vi "Write Message.vi"(8 "error in (no error)":errorcluster, 10 "Message":string, 11 "Printf_Msg_General in":refnum<class "LV_Printf Msg.lvclass">) -> (0 "error out":errorcluster, 3 "Printf_Msg_General out":refnum<class "LV_Printf Msg.lvclass">)   [LabVIEW 2013, in "SET_Printf.lvlib" / "LV_Printf Msg.lvclass"]
uses:
  LV_Printf Msg.lvclass
  LV_Printf Msg.lvclass/LV_Printf Msg.ctl
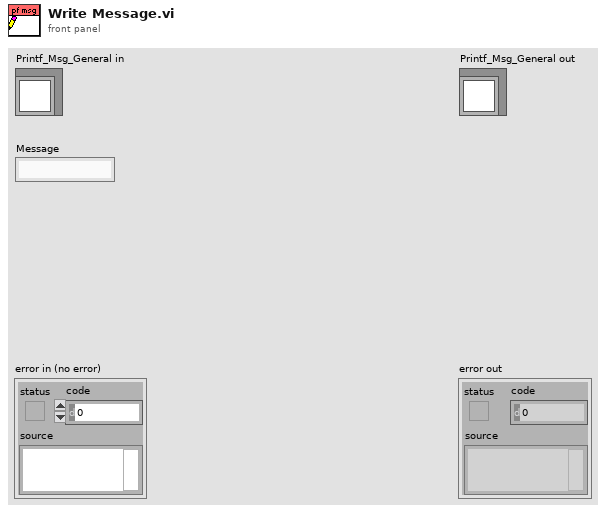
[diagram p1: front panel]
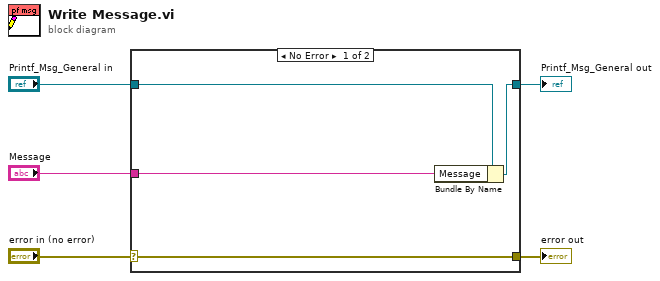
[diagram p0: block diagram]
diagram:
  n1 = case shown="No Error" "error in (no error)" {
    selector: "error in (no error)" -> [w9 w10]
    tunnel: [w9 w10] -> w4
    tunnel: [w7 w11] -> w2
    tunnel: "Printf_Msg_General in" -> [w8 w11]
    tunnel: "Message" -> [w6 _]
    frame No Error {
      n2 = Bundle By Name(cluster=w8, "Message"=w6) -> (w7:refnum<class "LV_Printf Msg.lvclass">)
    }
    frame Error {
    }
  }
  "error out" <- w4
  "Printf_Msg_General out" <- w2
